vi "micUnbundle_IV.vi"(0 "405nm Data":T3, 5 "532nm Data":T4, 7 "660nm Data":T5, 9 "785nm Data":T2) -> (4 "pd ts":T1(graph), 6 "405 New Array":dbl[](array[numeric]), 8 "532 New Array":dbl[](array[numeric]), 10 "660 New Array":dbl[](array[numeric]), 15 "785 New Array":dbl[](array[numeric]))   [LabVIEW 2011]
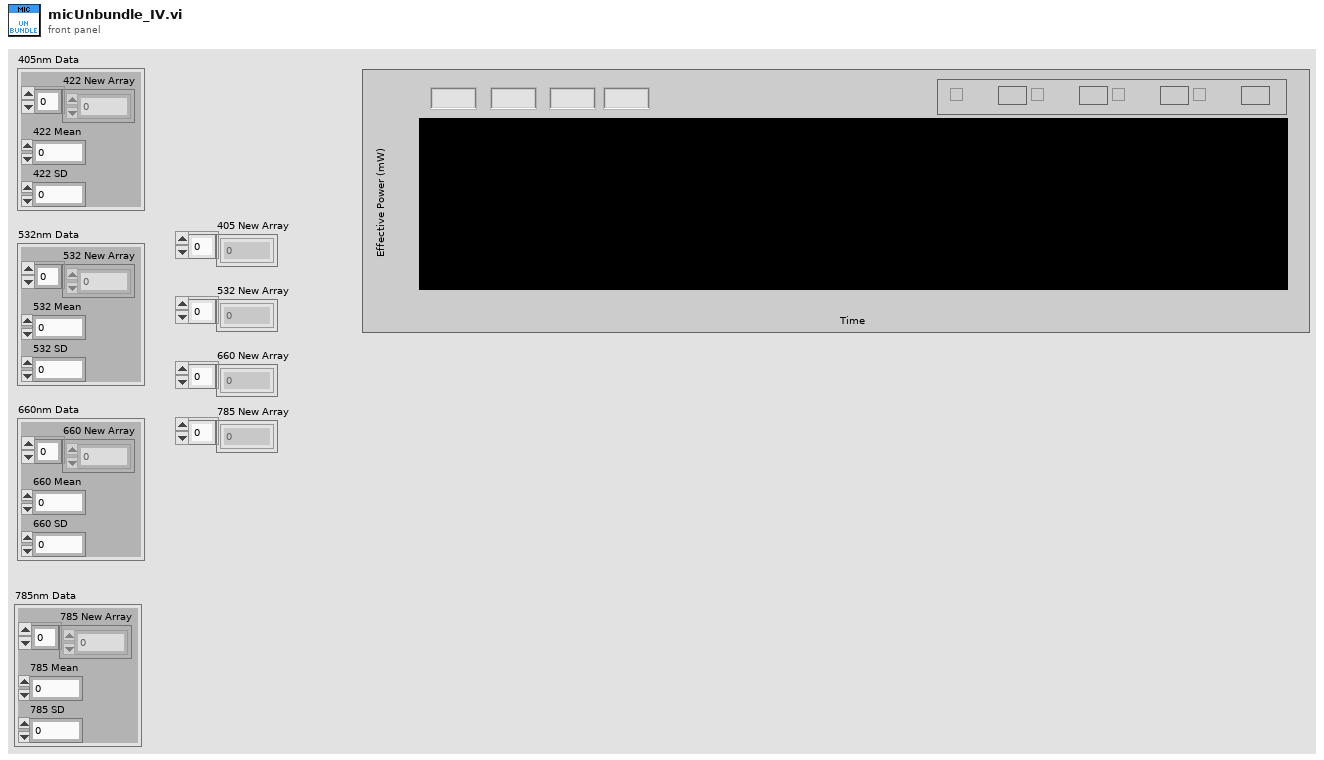
[diagram p1: front panel]
types:
  T1 = cluster{"422 Mean":dbl, "532 Mean":dbl, "660 Mean":dbl, "785 Mean":dbl}
  T2 = cluster{"785 New Array":dbl[], "785 Mean":dbl, "785 SD":dbl}
  T3 = cluster{"422 New Array":dbl[], "422 Mean":dbl, "422 SD":dbl}
  T4 = cluster{"532 New Array":dbl[], "532 Mean":dbl, "532 SD":dbl}
  T5 = cluster{"660 New Array":dbl[], "660 Mean":dbl, "660 SD":dbl}
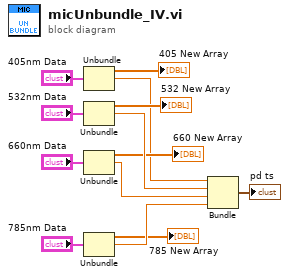
[diagram p0: block diagram]
diagram:
  n1 = Unbundle("405nm Data") -> ("422 New Array"=→"405 New Array":dbl[], "422 Mean"=w2:dbl)  [unwired: 1 out]
  n2 = Unbundle("532nm Data") -> ("532 New Array"=→"532 New Array":dbl[], "532 Mean"=w10:dbl)  [unwired: 1 out]
  n3 = Unbundle("660nm Data") -> ("660 New Array"=→"660 New Array":dbl[], "660 Mean"=w1:dbl)  [unwired: 1 out]
  n4 = Unbundle("785nm Data") -> ("785 New Array"=→"785 New Array":dbl[], "785 Mean"=w4:dbl)  [unwired: 1 out]
  n5 = Bundle("422 Mean"=w2, "532 Mean"=w10, "660 Mean"=w1, "785 Mean"=w4) -> (→"pd ts":T1)  [unwired: 1 in]
